vi "Defaults.vi"(8 "error in (no error)":errorcluster) -> (0 "error out":errorcluster)   [LabVIEW 2021, in "HttpServer.lvlib"]
uses:
  HttpServer.lvlib
  Page.vit
  Page Log.vi
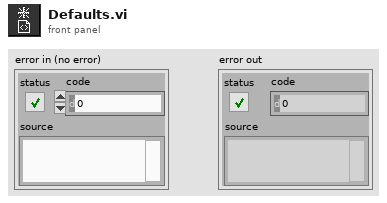
[diagram p1: front panel]
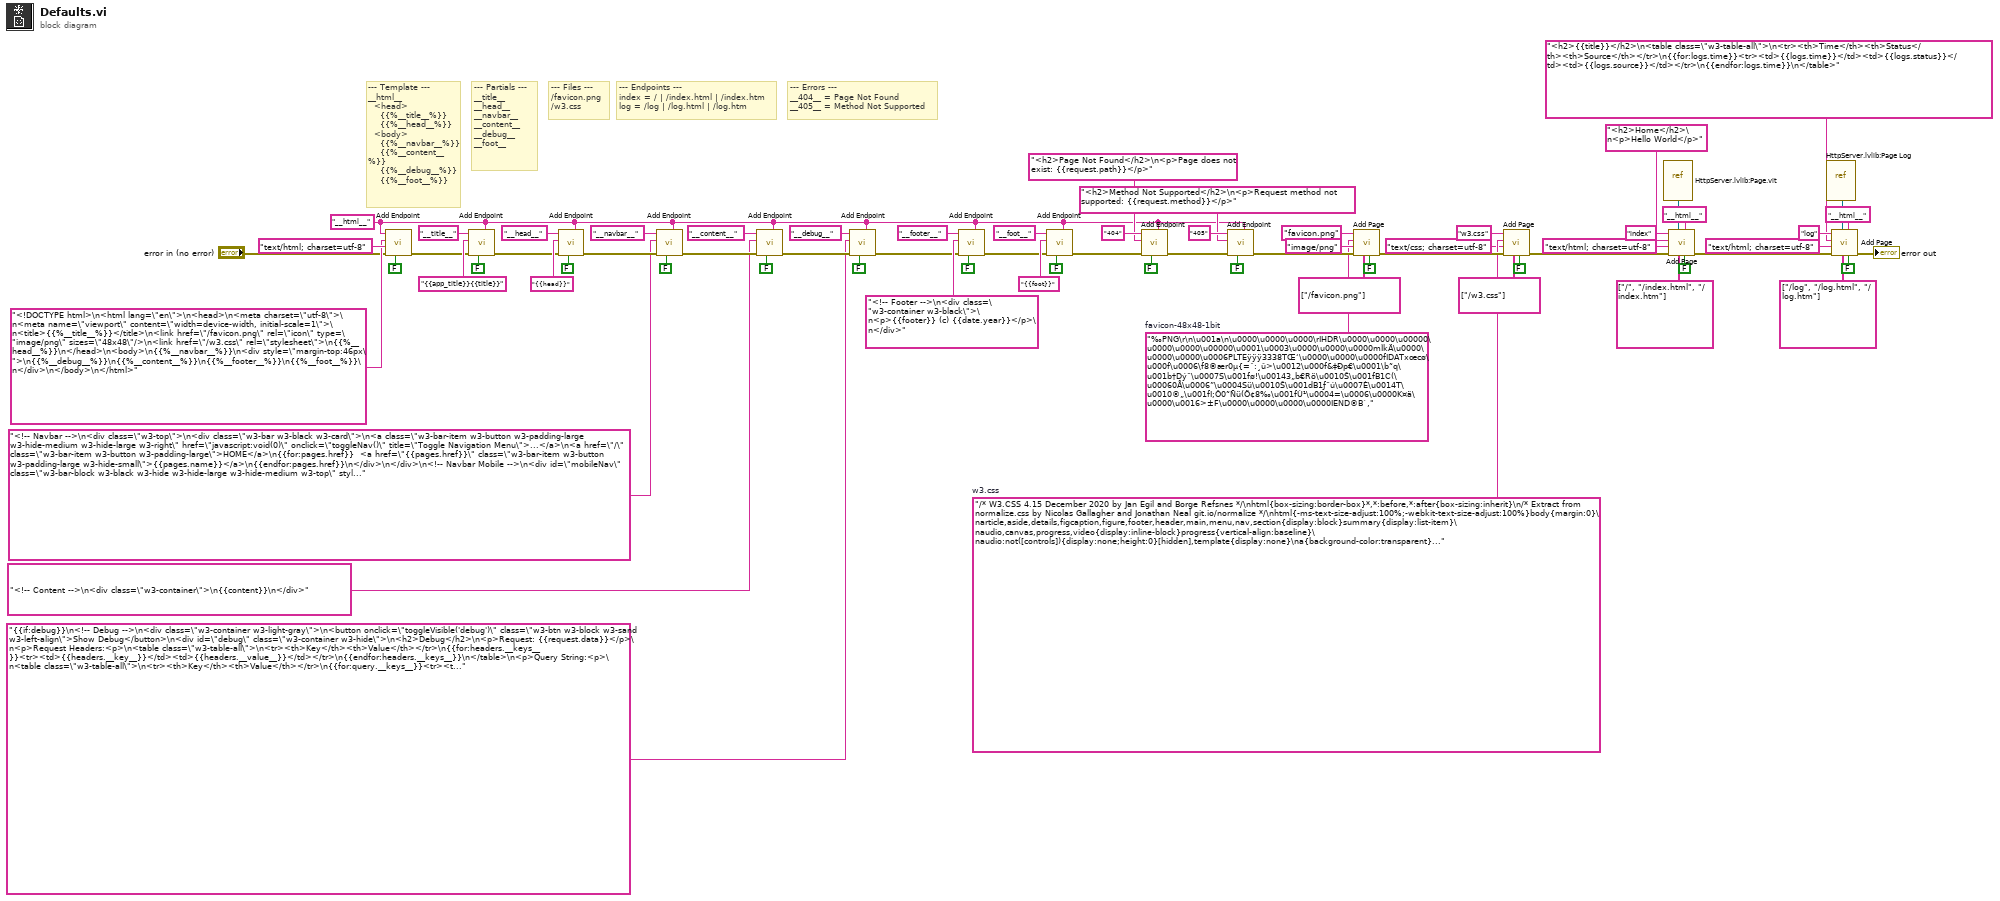
[diagram p0: block diagram]
diagram:
  w28 = "/* W3.CSS 4.15 December 2020 by Jan Egil and Borge Refsnes */\nhtml{box-sizing:border-box}*,*:before,*:after{box-sizing:inherit}\n/* Extract from normalize.css by Nicolas Gallagher and Jonathan Neal git.io/normalize */\nhtml{-ms-text-size-adjust:100%;-webkit-text-size-adjust:100%}body{margin:0}\narticle,aside,details,figcaption,figure,footer,header,main,menu,nav,section{display:block}summary{display:list-item}\naudio,canvas,progress,video{display:inline-block}progress{vertical-align:baseline}\naudio:not([controls]){display:none;height:0}[hidden],template{display:none}\na{background-color:transparent}a:active,a:hover{outline-width:0}\nabbr[title]{border-bottom:none;text-decoration:underline;text-decoration:underline dotted}\nb,strong{font-weight:bolder}dfn{font-style:italic}mark{background:#ff0;color:#000}\nsmall{font-size:80%}sub,sup{font-size:75%;line-height:0;position:relative;vertical-align:baseline}\nsub{bottom:-0.25em}sup{top:-0.5em}figure{margin:1em 40px}img{border-style:none}\ncode,kbd,pre,samp{font-family:monospace,monospace;font-size:1em}hr{box-sizing:content-box;height:0;overflow:visible}\nbutton,input,select,textarea,optgroup{font:inherit;margin:0}optgroup{font-weight:bold}\nbutton,input{overflow:visible}button,select{text-transform:none}\nbutton,[type=button],[type=reset],[type=submit]{-webkit-appearance:button}\nbutton::-moz-focus-inner,[type=button]::-moz-focus-inner,[type=reset]::-moz-focus-inner,[type=submit]::-moz-focus-inner{border-style:none;padding:0}\nbutton:-moz-focusring,[type=button]:-moz-focusring,[type=reset]:-moz-focusring,[type=submit]:-moz-focusring{outline:1px dotted ButtonText}\nfieldset{border:1px solid #c0c0c0;margin:0 2px;padding:.35em .625em .75em}\nlegend{color:inherit;display:table;max-width:100%;padding:0;white-space:normal}textarea{overflow:auto}\n[type=checkbox],[type=radio]{padding:0}\n[type=number]::-webkit-inner-spin-button,[type=number]::-webkit-outer-spin-button{height:auto}\n[type=search]{-webkit-appearance:textfield;outline-offset:-2px}\n[type=search]::-webkit-search-decoration{-webkit-appearance:none}\n::-webkit-file-upload-button{-webkit-appearance:button;font:inherit}\n/* End extract */\nhtml,body{font-family:Verdana,sans-serif;font-size:15px;line-height:1.5}html{overflow-x:hidden}\nh1{font-size:36px}h2{font-size:30px}h3{font-size:24px}h4{font-size:20px}h5{font-size:18px}h6{font-size:16px}\n.w3-serif{font-family:serif}.w3-sans-serif{font-family:sans-serif}.w3-cursive{font-family:cursive}.w3-monospace{font-family:monospace}\nh1,h2,h3,h4,h5,h6{font-family:\"Segoe UI\",Arial,sans-serif;font-weight:400;margin:10px 0}.w3-wide{letter-spacing:4px}\nhr{border:0;border-top:1px solid #eee;margin:20px 0}\n.w3-image{max-width:100%;height:auto}img{vertical-align:middle}a{color:inherit}\n.w3-table,.w3-table-all{border-collapse:collapse;border-spacing:0;width:100%;display:table}.w3-table-all{border:1px solid #ccc}\n.w3-bordered tr,.w3-table-all tr{border-bottom:1px solid #ddd}.w3-striped tbody tr:nth-child(even){background-color:#f1f1f1}\n.w3-table-all tr:nth-child(odd){background-color:#fff}.w3-table-all tr:nth-child(even){background-color:#f1f1f1}\n.w3-hoverable tbody tr:hover,.w3-ul.w3-hoverable li:hover{background-color:#ccc}.w3-centered tr th,.w3-centered tr td{text-align:center}\n.w3-table td,.w3-table th,.w3-table-all td,.w3-table-all th{padding:8px 8px;display:table-cell;text-align:left;vertical-align:top}\n.w3-table th:first-child,.w3-table td:first-child,.w3-table-all th:first-child,.w3-table-all td:first-child{padding-left:16px}\n.w3-btn,.w3-button{border:none;display:inline-block;padding:8px 16px;vertical-align:middle;overflow:hidden;text-decoration:none;color:inherit;background-color:inherit;text-align:center;cursor:pointer;white-space:nowrap}\n.w3-btn:hover{box-shadow:0 8px 16px 0 rgba(0,0,0,0.2),0 6px 20px 0 rgba(0,0,0,0.19)}\n.w3-btn,.w3-button{-webkit-touch-callout:none;-webkit-user-select:none;-khtml-user-select:none;-moz-user-select:none;-ms-user-select:none;user-select:none}   \n.w3-disabled,.w3-btn:disabled,.w3-button:disabled{cursor:not-allowed;opacity:0.3}.w3-disabled *,:disabled *{pointer-events:none}\n.w3-btn.w3-disabled:hover,.w3-btn:disabled:hover{box-shadow:none}\n.w3-badge,.w3-tag{background-color:#000;color:#fff;display:inline-block;padding-left:8px;padding-right:8px;text-align:center}.w3-badge{border-radius:50%}\n.w3-ul{list-style-type:none;padding:0;margin:0}.w3-ul li{padding:8px 16px;border-bottom:1px solid #ddd}.w3-ul li:last-child{border-bottom:none}\n.w3-tooltip,.w3-display-container{position:relative}.w3-tooltip .w3-text{display:none}.w3-tooltip:hover .w3-text{display:inline-block}\n.w3-ripple:active{opacity:0.5}.w3-ripple{transition:opacity 0s}\n.w3-input{padding:8px;display:block;border:none;border-bottom:1px solid #ccc;width:100%}\n.w3-select{padding:9px 0;width:100%;border:none;border-bottom:1px solid #ccc}\n.w3-dropdown-click,.w3-dropdown-hover{position:relative;display:inline-block;cursor:pointer}\n.w3-dropdown-hover:hover .w3-dropdown-content{display:block}\n.w3-dropdown-hover:first-child,.w3-dropdown-click:hover{background-color:#ccc;color:#000}\n.w3-dropdown-hover:hover > .w3-button:first-child,.w3-dropdown-click:hover > .w3-button:first-child{background-color:#ccc;color:#000}\n.w3-dropdown-content{cursor:auto;color:#000;background-color:#fff;display:none;position:absolute;min-width:160px;margin:0;padding:0;z-index:1}\n.w3-check,.w3-radio{width:24px;height:24px;position:relative;top:6px}\n.w3-sidebar{height:100%;width:200px;background-color:#fff;position:fixed!important;z-index:1;overflow:auto}\n.w3-bar-block .w3-dropdown-hover,.w3-bar-block .w3-dropdown-click{width:100%}\n.w3-bar-block .w3-dropdown-hover .w3-dropdown-content,.w3-bar-block .w3-dropdown-click .w3-dropdown-content{min-width:100%}\n.w3-bar-block .w3-dropdown-hover .w3-button,.w3-bar-block .w3-dropdown-click .w3-button{width:100%;text-align:left;padding:8px 16px}\n.w3-main,#main{transition:margin-left .4s}\n.w3-modal{z-index:3;display:none;padding-top:100px;position:fixed;left:0;top:0;width:100%;height:100%;overflow:auto;background-color:rgb(0,0,0);background-color:rgba(0,0,0,0.4)}\n.w3-modal-content{margin:auto;background-color:#fff;position:relative;padding:0;outline:0;width:600px}\n.w3-bar{width:100%;overflow:hidden}.w3-center .w3-bar{display:inline-block;width:auto}\n.w3-bar .w3-bar-item{padding:8px 16px;float:left;width:auto;border:none;display:block;outline:0}\n.w3-bar .w3-dropdown-hover,.w3-bar .w3-dropdown-click{position:static;float:left}\n.w3-bar .w3-button{white-space:normal}\n.w3-bar-block .w3-bar-item{width:100%;display:block;padding:8px 16px;text-align:left;border:none;white-space:normal;float:none;outline:0}\n.w3-bar-block.w3-center .w3-bar-item{text-align:center}.w3-block{display:block;width:100%}\n.w3-responsive{display:block;overflow-x:auto}\n.w3-container:after,.w3-container:before,.w3-panel:after,.w3-panel:before,.w3-row:after,.w3-row:before,.w3-row-padding:after,.w3-row-padding:before,\n.w3-cell-row:before,.w3-cell-row:after,.w3-clear:after,.w3-clear:before,.w3-bar:before,.w3-bar:after{content:\"\";display:table;clear:both}\n.w3-col,.w3-half,.w3-third,.w3-twothird,.w3-threequarter,.w3-quarter{float:left;width:100%}\n.w3-col.s1{width:8.33333%}.w3-col.s2{width:16.66666%}.w3-col.s3{width:24.99999%}.w3-col.s4{width:33.33333%}\n.w3-col.s5{width:41.66666%}.w3-col.s6{width:49.99999%}.w3-col.s7{width:58.33333%}.w3-col.s8{width:66.66666%}\n.w3-col.s9{width:74.99999%}.w3-col.s10{width:83.33333%}.w3-col.s11{width:91.66666%}.w3-col.s12{width:99.99999%}\n@media (min-width:601px){.w3-col.m1{width:8.33333%}.w3-col.m2{width:16.66666%}.w3-col.m3,.w3-quarter{width:24.99999%}.w3-col.m4,.w3-third{width:33.33333%}\n.w3-col.m5{width:41.66666%}.w3-col.m6,.w3-half{width:49.99999%}.w3-col.m7{width:58.33333%}.w3-col.m8,.w3-twothird{width:66.66666%}\n.w3-col.m9,.w3-threequarter{width:74.99999%}.w3-col.m10{width:83.33333%}.w3-col.m11{width:91.66666%}.w3-col.m12{width:99.99999%}}\n@media (min-width:993px){.w3-col.l1{width:8.33333%}.w3-col.l2{width:16.66666%}.w3-col.l3{width:24.99999%}.w3-col.l4{width:33.33333%}\n.w3-col.l5{width:41.66666%}.w3-col.l6{width:49.99999%}.w3-col.l7{width:58.33333%}.w3-col.l8{width:66.66666%}\n.w3-col.l9{width:74.99999%}.w3-col.l10{width:83.33333%}.w3-col.l11{width:91.66666%}.w3-col.l12{width:99.99999%}}\n.w3-rest{overflow:hidden}.w3-stretch{margin-left:-16px;margin-right:-16px}\n.w3-content,.w3-auto{margin-left:auto;margin-right:auto}.w3-content{max-width:980px}.w3-auto{max-width:1140px}\n.w3-cell-row{display:table;width:100%}.w3-cell{display:table-cell}\n.w3-cell-top{vertical-align:top}.w3-cell-middle{vertical-align:middle}.w3-cell-bottom{vertical-align:bottom}\n.w3-hide{display:none!important}.w3-show-block,.w3-show{display:block!important}.w3-show-inline-block{display:inline-block!important}\n@media (max-width:1205px){.w3-auto{max-width:95%}}\n@media (max-width:600px){.w3-modal-content{margin:0 10px;width:auto!important}.w3-modal{padding-top:30px}\n.w3-dropdown-hover.w3-mobile .w3-dropdown-content,.w3-dropdown-click.w3-mobile .w3-dropdown-content{position:relative}\t\n.w3-hide-small{display:none!important}.w3-mobile{display:block;width:100%!important}.w3-bar-item.w3-mobile,.w3-dropdown-hover.w3-mobile,.w3-dropdown-click.w3-mobile{text-align:center}\n.w3-dropdown-hover.w3-mobile,.w3-dropdown-hover.w3-mobile .w3-btn,.w3-dropdown-hover.w3-mobile .w3-button,.w3-dropdown-click.w3-mobile,.w3-dropdown-click.w3-mobile .w3-btn,.w3-dropdown-click.w3-mobile .w3-button{width:100%}}\n@media (max-width:768px){.w3-modal-content{width:500px}.w3-modal{padding-top:50px}}\n@media (min-width:993px){.w3-modal-content{width:900px}.w3-hide-large{display:none!important}.w3-sidebar.w3-collapse{display:block!important}}\n@media (max-width:992px) and (min-width:601px){.w3-hide-medium{display:none!important}}\n@media (max-width:992px){.w3-sidebar.w3-collapse{display:none}.w3-main{margin-left:0!important;margin-right:0!important}.w3-auto{max-width:100%}}\n.w3-top,.w3-bottom{position:fixed;width:100%;z-index:1}.w3-top{top:0}.w3-bottom{bottom:0}\n.w3-overlay{position:fixed;display:none;width:100%;height:100%;top:0;left:0;right:0;bottom:0;background-color:rgba(0,0,0,0.5);z-index:2}\n.w3-display-topleft{position:absolute;left:0;top:0}.w3-display-topright{position:absolute;right:0;top:0}\n.w3-display-bottomleft{position:absolute;left:0;bottom:0}.w3-display-bottomright{position:absolute;right:0;bottom:0}\n.w3-display-middle{position:absolute;top:50%;left:50%;transform:translate(-50%,-50%);-ms-transform:translate(-50%,-50%)}\n.w3-display-left{position:absolute;top:50%;left:0%;transform:translate(0%,-50%);-ms-transform:translate(-0%,-50%)}\n.w3-display-right{position:absolute;top:50%;right:0%;transform:translate(0%,-50%);-ms-transform:translate(0%,-50%)}\n.w3-display-topmiddle{position:absolute;left:50%;top:0;transform:translate(-50%,0%);-ms-transform:translate(-50%,0%)}\n.w3-display-bottommiddle{position:absolute;left:50%;bottom:0;transform:translate(-50%,0%);-ms-transform:translate(-50%,0%)}\n.w3-display-container:hover .w3-display-hover{display:block}.w3-display-container:hover span.w3-display-hover{display:inline-block}.w3-display-hover{display:none}\n.w3-display-position{position:absolute}\n.w3-circle{border-radius:50%}\n.w3-round-small{border-radius:2px}.w3-round,.w3-round-medium{border-radius:4px}.w3-round-large{border-radius:8px}.w3-round-xlarge{border-radius:16px}.w3-round-xxlarge{border-radius:32px}\n.w3-row-padding,.w3-row-padding>.w3-half,.w3-row-padding>.w3-third,.w3-row-padding>.w3-twothird,.w3-row-padding>.w3-threequarter,.w3-row-padding>.w3-quarter,.w3-row-padding>.w3-col{padding:0 8px}\n.w3-container,.w3-panel{padding:0.01em 16px}.w3-panel{margin-top:16px;margin-bottom:16px}\n.w3-code,.w3-codespan{font-family:Consolas,\"courier new\";font-size:16px}\n.w3-code{width:auto;background-color:#fff;padding:8px 12px;border-left:4px solid #4CAF50;word-wrap:break-word}\n.w3-codespan{color:crimson;background-color:#f1f1f1;padding-left:4px;padding-right:4px;font-size:110%}\n.w3-card,.w3-card-2{box-shadow:0 2px 5px 0 rgba(0,0,0,0.16),0 2px 10px 0 rgba(0,0,0,0.12)}\n.w3-card-4,.w3-hover-shadow:hover{box-shadow:0 4px 10px 0 rgba(0,0,0,0.2),0 4px 20px 0 rgba(0,0,0,0.19)}\n.w3-spin{animation:w3-spin 2s infinite linear}@keyframes w3-spin{0%{transform:rotate(0deg)}100%{transform:rotate(359deg)}}\n.w3-animate-fading{animation:fading 10s infinite}@keyframes fading{0%{opacity:0}50%{opacity:1}100%{opacity:0}}\n.w3-animate-opacity{animation:opac 0.8s}@keyframes opac{from{opacity:0} to{opacity:1}}\n.w3-animate-top{position:relative;animation:animatetop 0.4s}@keyframes animatetop{from{top:-300px;opacity:0} to{top:0;opacity:1}}\n.w3-animate-left{position:relative;animation:animateleft 0.4s}@keyframes animateleft{from{left:-300px;opacity:0} to{left:0;opacity:1}}\n.w3-animate-right{position:relative;animation:animateright 0.4s}@keyframes animateright{from{right:-300px;opacity:0} to{right:0;opacity:1}}\n.w3-animate-bottom{position:relative;animation:animatebottom 0.4s}@keyframes animatebottom{from{bottom:-300px;opacity:0} to{bottom:0;opacity:1}}\n.w3-animate-zoom {animation:animatezoom 0.6s}@keyframes animatezoom{from{transform:scale(0)} to{transform:scale(1)}}\n.w3-animate-input{transition:width 0.4s ease-in-out}.w3-animate-input:focus{width:100%!important}\n.w3-opacity,.w3-hover-opacity:hover{opacity:0.60}.w3-opacity-off,.w3-hover-opacity-off:hover{opacity:1}\n.w3-opacity-max{opacity:0.25}.w3-opacity-min{opacity:0.75}\n.w3-greyscale-max,.w3-grayscale-max,.w3-hover-greyscale:hover,.w3-hover-grayscale:hover{filter:grayscale(100%)}\n.w3-greyscale,.w3-grayscale{filter:grayscale(75%)}.w3-greyscale-min,.w3-grayscale-min{filter:grayscale(50%)}\n.w3-sepia{filter:sepia(75%)}.w3-sepia-max,.w3-hover-sepia:hover{filter:sepia(100%)}.w3-sepia-min{filter:sepia(50%)}\n.w3-tiny{font-size:10px!important}.w3-small{font-size:12px!important}.w3-medium{font-size:15px!important}.w3-large{font-size:18px!important}\n.w3-xlarge{font-size:24px!important}.w3-xxlarge{font-size:36px!important}.w3-xxxlarge{font-size:48px!important}.w3-jumbo{font-size:64px!important}\n.w3-left-align{text-align:left!important}.w3-right-align{text-align:right!important}.w3-justify{text-align:justify!important}.w3-center{text-align:center!important}\n.w3-border-0{border:0!important}.w3-border{border:1px solid #ccc!important}\n.w3-border-top{border-top:1px solid #ccc!important}.w3-border-bottom{border-bottom:1px solid #ccc!important}\n.w3-border-left{border-left:1px solid #ccc!important}.w3-border-right{border-right:1px solid #ccc!important}\n.w3-topbar{border-top:6px solid #ccc!important}.w3-bottombar{border-bottom:6px solid #ccc!important}\n.w3-leftbar{border-left:6px solid #ccc!important}.w3-rightbar{border-right:6px solid #ccc!important}\n.w3-section,.w3-code{margin-top:16px!important;margin-bottom:16px!important}\n.w3-margin{margin:16px!important}.w3-margin-top{margin-top:16px!important}.w3-margin-bottom{margin-bottom:16px!important}\n.w3-margin-left{margin-left:16px!important}.w3-margin-right{margin-right:16px!important}\n.w3-padding-small{padding:4px 8px!important}.w3-padding{padding:8px 16px!important}.w3-padding-large{padding:12px 24px!important}\n.w3-padding-16{padding-top:16px!important;padding-bottom:16px!important}.w3-padding-24{padding-top:24px!important;padding-bottom:24px!important}\n.w3-padding-32{padding-top:32px!important;padding-bottom:32px!important}.w3-padding-48{padding-top:48px!important;padding-bottom:48px!important}\n.w3-padding-64{padding-top:64px!important;padding-bottom:64px!important}\n.w3-padding-top-64{padding-top:64px!important}.w3-padding-top-48{padding-top:48px!important}\n.w3-padding-top-32{padding-top:32px!important}.w3-padding-top-24{padding-top:24px!important}\n.w3-left{float:left!important}.w3-right{float:right!important}\n.w3-button:hover{color:#000!important;background-color:#ccc!important}\n.w3-transparent,.w3-hover-none:hover{background-color:transparent!important}\n.w3-hover-none:hover{box-shadow:none!important}\n/* Colors */\n.w3-amber,.w3-hover-amber:hover{color:#000!important;background-color:#ffc107!important}\n.w3-aqua,.w3-hover-aqua:hover{color:#000!important;background-color:#00ffff!important}\n.w3-blue,.w3-hover-blue:hover{color:#fff!important;background-color:#2196F3!important}\n.w3-light-blue,.w3-hover-light-blue:hover{color:#000!important;background-color:#87CEEB!important}\n.w3-brown,.w3-hover-brown:hover{color:#fff!important;background-color:#795548!important}\n.w3-cyan,.w3-hover-cyan:hover{color:#000!important;background-color:#00bcd4!important}\n.w3-blue-grey,.w3-hover-blue-grey:hover,.w3-blue-gray,.w3-hover-blue-gray:hover{color:#fff!important;background-color:#607d8b!important}\n.w3-green,.w3-hover-green:hover{color:#fff!important;background-color:#4CAF50!important}\n.w3-light-green,.w3-hover-light-green:hover{color:#000!important;background-color:#8bc34a!important}\n.w3-indigo,.w3-hover-indigo:hover{color:#fff!important;background-color:#3f51b5!important}\n.w3-khaki,.w3-hover-khaki:hover{color:#000!important;background-color:#f0e68c!important}\n.w3-lime,.w3-hover-lime:hover{color:#000!important;background-color:#cddc39!important}\n.w3-orange,.w3-hover-orange:hover{color:#000!important;background-color:#ff9800!important}\n.w3-deep-orange,.w3-hover-deep-orange:hover{color:#fff!important;background-color:#ff5722!important}\n.w3-pink,.w3-hover-pink:hover{color:#fff!important;background-color:#e91e63!important}\n.w3-purple,.w3-hover-purple:hover{color:#fff!important;background-color:#9c27b0!important}\n.w3-deep-purple,.w3-hover-deep-purple:hover{color:#fff!important;background-color:#673ab7!important}\n.w3-red,.w3-hover-red:hover{color:#fff!important;background-color:#f44336!important}\n.w3-sand,.w3-hover-sand:hover{color:#000!important;background-color:#fdf5e6!important}\n.w3-teal,.w3-hover-teal:hover{color:#fff!important;background-color:#009688!important}\n.w3-yellow,.w3-hover-yellow:hover{color:#000!important;background-color:#ffeb3b!important}\n.w3-white,.w3-hover-white:hover{color:#000!important;background-color:#fff!important}\n.w3-black,.w3-hover-black:hover{color:#fff!important;background-color:#000!important}\n.w3-grey,.w3-hover-grey:hover,.w3-gray,.w3-hover-gray:hover{color:#000!important;background-color:#9e9e9e!important}\n.w3-light-grey,.w3-hover-light-grey:hover,.w3-light-gray,.w3-hover-light-gray:hover{color:#000!important;background-color:#f1f1f1!important}\n.w3-dark-grey,.w3-hover-dark-grey:hover,.w3-dark-gray,.w3-hover-dark-gray:hover{color:#fff!important;background-color:#616161!important}\n.w3-pale-red,.w3-hover-pale-red:hover{color:#000!important;background-color:#ffdddd!important}\n.w3-pale-green,.w3-hover-pale-green:hover{color:#000!important;background-color:#ddffdd!important}\n.w3-pale-yellow,.w3-hover-pale-yellow:hover{color:#000!important;background-color:#ffffcc!important}\n.w3-pale-blue,.w3-hover-pale-blue:hover{color:#000!important;background-color:#ddffff!important}\n.w3-text-amber,.w3-hover-text-amber:hover{color:#ffc107!important}\n.w3-text-aqua,.w3-hover-text-aqua:hover{color:#00ffff!important}\n.w3-text-blue,.w3-hover-text-blue:hover{color:#2196F3!important}\n.w3-text-light-blue,.w3-hover-text-light-blue:hover{color:#87CEEB!important}\n.w3-text-brown,.w3-hover-text-brown:hover{color:#795548!important}\n.w3-text-cyan,.w3-hover-text-cyan:hover{color:#00bcd4!important}\n.w3-text-blue-grey,.w3-hover-text-blue-grey:hover,.w3-text-blue-gray,.w3-hover-text-blue-gray:hover{color:#607d8b!important}\n.w3-text-green,.w3-hover-text-green:hover{color:#4CAF50!important}\n.w3-text-light-green,.w3-hover-text-light-green:hover{color:#8bc34a!important}\n.w3-text-indigo,.w3-hover-text-indigo:hover{color:#3f51b5!important}\n.w3-text-khaki,.w3-hover-text-khaki:hover{color:#b4aa50!important}\n.w3-text-lime,.w3-hover-text-lime:hover{color:#cddc39!important}\n.w3-text-orange,.w3-hover-text-orange:hover{color:#ff9800!important}\n.w3-text-deep-orange,.w3-hover-text-deep-orange:hover{color:#ff5722!important}\n.w3-text-pink,.w3-hover-text-pink:hover{color:#e91e63!important}\n.w3-text-purple,.w3-hover-text-purple:hover{color:#9c27b0!important}\n.w3-text-deep-purple,.w3-hover-text-deep-purple:hover{color:#673ab7!important}\n.w3-text-red,.w3-hover-text-red:hover{color:#f44336!important}\n.w3-text-sand,.w3-hover-text-sand:hover{color:#fdf5e6!important}\n.w3-text-teal,.w3-hover-text-teal:hover{color:#009688!important}\n.w3-text-yellow,.w3-hover-text-yellow:hover{color:#d2be0e!important}\n.w3-text-white,.w3-hover-text-white:hover{color:#fff!important}\n.w3-text-black,.w3-hover-text-black:hover{color:#000!important}\n.w3-text-grey,.w3-hover-text-grey:hover,.w3-text-gray,.w3-hover-text-gray:hover{color:#757575!important}\n.w3-text-light-grey,.w3-hover-text-light-grey:hover,.w3-text-light-gray,.w3-hover-text-light-gray:hover{color:#f1f1f1!important}\n.w3-text-dark-grey,.w3-hover-text-dark-grey:hover,.w3-text-dark-gray,.w3-hover-text-dark-gray:hover{color:#3a3a3a!important}\n.w3-border-amber,.w3-hover-border-amber:hover{border-color:#ffc107!important}\n.w3-border-aqua,.w3-hover-border-aqua:hover{border-color:#00ffff!important}\n.w3-border-blue,.w3-hover-border-blue:hover{border-color:#2196F3!important}\n.w3-border-light-blue,.w3-hover-border-light-blue:hover{border-color:#87CEEB!important}\n.w3-border-brown,.w3-hover-border-brown:hover{border-color:#795548!important}\n.w3-border-cyan,.w3-hover-border-cyan:hover{border-color:#00bcd4!important}\n.w3-border-blue-grey,.w3-hover-border-blue-grey:hover,.w3-border-blue-gray,.w3-hover-border-blue-gray:hover{border-color:#607d8b!important}\n.w3-border-green,.w3-hover-border-green:hover{border-color:#4CAF50!important}\n.w3-border-light-green,.w3-hover-border-light-green:hover{border-color:#8bc34a!important}\n.w3-border-indigo,.w3-hover-border-indigo:hover{border-color:#3f51b5!important}\n.w3-border-khaki,.w3-hover-border-khaki:hover{border-color:#f0e68c!important}\n.w3-border-lime,.w3-hover-border-lime:hover{border-color:#cddc39!important}\n.w3-border-orange,.w3-hover-border-orange:hover{border-color:#ff9800!important}\n.w3-border-deep-orange,.w3-hover-border-deep-orange:hover{border-color:#ff5722!important}\n.w3-border-pink,.w3-hover-border-pink:hover{border-color:#e91e63!important}\n.w3-border-purple,.w3-hover-border-purple:hover{border-color:#9c27b0!important}\n.w3-border-deep-purple,.w3-hover-border-deep-purple:hover{border-color:#673ab7!important}\n.w3-border-red,.w3-hover-border-red:hover{border-color:#f44336!important}\n.w3-border-sand,.w3-hover-border-sand:hover{border-color:#fdf5e6!important}\n.w3-border-teal,.w3-hover-border-teal:hover{border-color:#009688!important}\n.w3-border-yellow,.w3-hover-border-yellow:hover{border-color:#ffeb3b!important}\n.w3-border-white,.w3-hover-border-white:hover{border-color:#fff!important}\n.w3-border-black,.w3-hover-border-black:hover{border-color:#000!important}\n.w3-border-grey,.w3-hover-border-grey:hover,.w3-border-gray,.w3-hover-border-gray:hover{border-color:#9e9e9e!important}\n.w3-border-light-grey,.w3-hover-border-light-grey:hover,.w3-border-light-gray,.w3-hover-border-light-gray:hover{border-color:#f1f1f1!important}\n.w3-border-dark-grey,.w3-hover-border-dark-grey:hover,.w3-border-dark-gray,.w3-hover-border-dark-gray:hover{border-color:#616161!important}\n.w3-border-pale-red,.w3-hover-border-pale-red:hover{border-color:#ffe7e7!important}.w3-border-pale-green,.w3-hover-border-pale-green:hover{border-color:#e7ffe7!important}\n.w3-border-pale-yellow,.w3-hover-border-pale-yellow:hover{border-color:#ffffcc!important}.w3-border-pale-blue,.w3-hover-border-pale-blue:hover{border-color:#e7ffff!important}\n"  # w3.css
  w33 = "‰PNG\r\n\u001a\n\u0000\u0000\u0000\rIHDR\u0000\u0000\u00000\u0000\u0000\u00000\u0001\u0003\u0000\u0000\u0000mÌkÄ\u0000\u0000\u0000\u0006PLTEÿÿÿ3338TŒ‘\u0000\u0000\u0000fIDATxœcø\u000f\u0006\f8©ær0µ{=ˆ:¸û>\u0012\u000f&‡Ðp€\u0001\b˜q\u001b†Dý¨\u0007S\u001fø!\u00143„b€Rö\u0010Š\u001fB1C(\u00060Å\u0006”\u0004Sü\u0010Š\u001dB1ƒ¨ú\u0007È\u0014T\u0010®„\u001fI;Ô0˜Ñü(Ö¢8‰\u001fÙ¹\u0004=\u0006\u0000K¤ä\u0000\u0016>±F\u0000\u0000\u0000\u0000IEND®B`‚"  # favicon-48x48-1bit
  w1 = "__html__" ("Template (\"\")")
  # "--- Partials ---\n__title__\n__head__\n__navbar__\n__content__\n__debug__\n__foot__"
  # "--- Errors ---\n__404__ = Page Not Found\n__405__ = Method Not Supported"
  # "--- Endpoints ---\nindex = / | /index.html | /index.htm\nlog = /log | /log.html | /log.htm"
  # "--- Template ---\n__html__\n  <head>\n    {{%__title__%}}\n    {{%__head__%}}\n  <body>\n    {{%__navbar__%}}\n    {{%__content__%}}\n    {{%__debug__%}}\n    {{%__foot__%}}"
  # "--- Files ---\n/favicon.png\n/w3.css"
  n1 = call "Add Endpoint.vi"("Replace if exists? (T)"=FALSE, "error in (no error)"="error in (no error)", "Content-Type"="text/html; charset=utf-8", "Content"="<!DOCTYPE html>\n<html lang=\"en\">\n<head>\n<meta charset=\"utf-8\">\n<meta name=\"viewport\" content=\"width=device-width, initial-scale=1\">\n<title>{{%__title__%}}</title>\n<link href=\"/favicon.png\" rel=\"icon\" type=\"image/png\" sizes=\"48x48\"/>\n<link href=\"/w3.css\" rel=\"stylesheet\">\n{{%__head__%}}\n</head>\n<body>\n{{%__navbar__%}}\n<div style=\"margin-top:46px\">\n{{%__debug__%}}\n{{%__content__%}}\n{{%__footer__%}}\n{{%__foot__%}}\n</div>\n</body>\n</html>", "Endpoint"=w1) -> ("error out"=w53:errorcluster)  [unwired: 5 in, 1 out]
  n2 = call "Add Endpoint.vi"("Template (\"\"=Static File)"=w1, "Replace if exists? (T)"=FALSE, "error in (no error)"=w53, "Content"="{{app_title}}{{title}}", "Endpoint"="__title__") -> ("error out"=w52:errorcluster)  [unwired: 5 in, 1 out]
  n3 = call "Add Endpoint.vi"("Template (\"\"=Static File)"=w1, "Replace if exists? (T)"=FALSE, "error in (no error)"=w52, "Content"="{{head}}", "Endpoint"="__head__") -> ("error out"=w51:errorcluster)  [unwired: 5 in, 1 out]
  n4 = call "Add Endpoint.vi"("Template (\"\"=Static File)"=w1, "Replace if exists? (T)"=FALSE, "error in (no error)"=w51, "Content"="<!-- Navbar -->\n<div class=\"w3-top\">\n<div class=\"w3-bar w3-black w3-card\">\n<a class=\"w3-bar-item w3-button w3-padding-large w3-hide-medium w3-hide-large w3-right\" href=\"javascript:void(0)\" onclick=\"toggleNav()\" title=\"Toggle Navigation Menu\">...</a>\n<a href=\"/\" class=\"w3-bar-item w3-button w3-padding-large\">HOME</a>\n{{for:pages.href}}  <a href=\"{{pages.href}}\" class=\"w3-bar-item w3-button w3-padding-large w3-hide-small\">{{pages.name}}</a>\n{{endfor:pages.href}}\n</div>\n</div>\n<!-- Navbar Mobile -->\n<div id=\"mobileNav\" class=\"w3-bar-block w3-black w3-hide w3-hide-large w3-hide-medium w3-top\" style=\"margin-top:46px\">\n{{for:pages.href}}  <a href=\"{{pages.href}}\" class=\"w3-bar-item w3-button w3-padding-large\" onclick=\"toggleNav()\">{{pages.name}}</a>\n{{endfor:pages.href}}\n</div>\n<script>\nfunction toggleNav() {\n  var x = document.getElementById(\"mobileNav\");\n  if (x.className.indexOf(\"w3-show\") == -1) { x.className += \" w3-show\"; } else { x.className = x.className.replace(\" w3-show\", \"\"); }\n}\n</script>", "Endpoint"="__navbar__") -> ("error out"=w48:errorcluster)  [unwired: 5 in, 1 out]
  n5 = call "Add Endpoint.vi"("Template (\"\"=Static File)"=w1, "Replace if exists? (T)"=FALSE, "error in (no error)"=w48, "Content"="<!-- Content -->\n<div class=\"w3-container\">\n{{content}}\n</div>", "Endpoint"="__content__") -> ("error out"=w43:errorcluster)  [unwired: 5 in, 1 out]
  n6 = call "Add Endpoint.vi"("Template (\"\"=Static File)"=w1, "Replace if exists? (T)"=FALSE, "error in (no error)"=w43, "Content"="{{if:debug}}\n<!-- Debug -->\n<div class=\"w3-container w3-light-gray\">\n<button onclick=\"toggleVisible('debug')\" class=\"w3-btn w3-block w3-sand w3-left-align\">Show Debug</button>\n<div id=\"debug\" class=\"w3-container w3-hide\">\n<h2>Debug</h2>\n<p>Request: {{request.data}}</p>\n<p>Request Headers:<p>\n<table class=\"w3-table-all\">\n<tr><th>Key</th><th>Value</th></tr>\n{{for:headers.__keys__}}<tr><td>{{headers.__key__}}</td><td>{{headers.__value__}}</td></tr>\n{{endfor:headers.__keys__}}\n</table>\n<p>Query String:<p>\n<table class=\"w3-table-all\">\n<tr><th>Key</th><th>Value</th></tr>\n{{for:query.__keys__}}<tr><td>{{query.__key__}}</td><td>{{query.__value__}}</td></tr>\n{{endfor:query.__keys__}}\n</table>\n<p>Form (POST Data):<p>\n<table class=\"w3-table-all\">\n<tr><th>Key</th><th>Value</th></tr>\n{{for:form.__keys__}}<tr><td>{{form.__key__}}</td><td>{{form.__value__}}</td></tr>\n{{endfor:form.__keys__}}\n</table>\n</div>\n</div>\n<script>\nfunction toggleVisible(id) {\n  var x = document.getElementById(id);\n  if (x.className.indexOf(\"w3-show\") == -1) {\n    x.className += \" w3-show\";\n  } else { \n    x.className = x.className.replace(\" w3-show\", \"\");\n  }\n}\n</script>\n{{endif:debug}}", "Endpoint"="__debug__") -> ("error out"=w3:errorcluster)  [unwired: 5 in, 1 out]
  n7 = call "Add Endpoint.vi"("Template (\"\"=Static File)"=w1, "Replace if exists? (T)"=FALSE, "error in (no error)"=w3, "Content"="<!-- Footer -->\n<div class=\"w3-container w3-black\">\n<p>{{footer}} (c) {{date.year}}</p>\n</div>", "Endpoint"="__footer__") -> ("error out"=w2:errorcluster)  [unwired: 5 in, 1 out]
  n8 = call "Add Endpoint.vi"("Template (\"\"=Static File)"=w1, "Replace if exists? (T)"=FALSE, "error in (no error)"=w2, "Content"="{{foot}}", "Endpoint"="__foot__") -> ("error out"=w38:errorcluster)  [unwired: 5 in, 1 out]
  n9 = call "Add Endpoint.vi"("Template (\"\"=Static File)"=w1, "Replace if exists? (T)"=FALSE ("Replace If Exists? (T)"), "error in (no error)"=w38, "Content"="<h2>Page Not Found</h2>\n<p>Page does not exist: {{request.path}}</p>", "Endpoint"="404") -> ("error out"=w37:errorcluster)  [unwired: 5 in, 1 out]
  n10 = call "Add Endpoint.vi"("Template (\"\"=Static File)"=w1, "Replace if exists? (T)"=FALSE, "error in (no error)"=w37, "Content"="<h2>Method Not Supported</h2>\n<p>Request method not supported: {{request.method}}</p>", "Endpoint"="405") -> ("error out"=w36:errorcluster)  [unwired: 5 in, 1 out]
  n11 = call "Add Page.vi"("Replace If Exists? (T)"=FALSE, "Paths"=string[] ["/favicon.png"], "error in (no error)"=w36, "Content-Type"="image/png" ("Content-Type in"), "Content"=w33, "Endpoint"="favicon.png" ("Uri")) -> ("error out"=w29:errorcluster)  [unwired: 5 in]
  n12 = call "Add Page.vi"("Replace If Exists? (T)"=FALSE, "Paths"=string[] ["/w3.css"], "error in (no error)"=w29, "Content-Type"="text/css; charset=utf-8", "Content"=w28, "Endpoint"="w3.css" ("Uri")) -> ("error out"=w20:errorcluster)  [unwired: 5 in]
  n13 = vi-ref "HttpServer.lvlib:Page.vit"() -> (w19:refnum<vi>)
  n14 = call "Add Page.vi"("Replace If Exists? (T)"=FALSE, "Template (\"\")"="__html__" ("Template (\"\")"), "Paths"=string[] ["/", "/index.html", "/index.htm"], "VI Refnum (NaN)"=w19, "error in (no error)"=w20, "Content-Type"="text/html; charset=utf-8", "Content"="<h2>Home</h2>\n<p>Hello World</p>", "Endpoint"="index" ("Uri")) -> ("error out"=w14:errorcluster)  [unwired: 3 in]
  n15 = vi-ref "HttpServer.lvlib:Page Log.vi"() -> (w18:refnum<vi>)
  n16 = call "Add Page.vi"("Replace If Exists? (T)"=FALSE, "Template (\"\")"="__html__" ("Template (\"\")"), "Paths"=string[] ["/log", "/log.html", "/log.htm"], "VI Refnum (NaN)"=w18, "error in (no error)"=w14, "Content-Type"="text/html; charset=utf-8", "Content"="<h2>{{title}}</h2>\n<table class=\"w3-table-all\">\n<tr><th>Time</th><th>Status</th><th>Source</th></tr>\n{{for:logs.time}}<tr><td>{{logs.time}}</td><td>{{logs.status}}</td><td>{{logs.source}}</td></tr>\n{{endfor:logs.time}}\n</table>", "Endpoint"="log" ("Uri")) -> ("error out"=→"error out":errorcluster)  [unwired: 3 in]
